vi "spectrometer-control.vi"(0 "Value Indicators Input":T3, 5 "Values changed":bool[](array[boolean]), 7 "Spectrograph Reset Input":T1, 8 "Reset Indicators after Init/Loop":T2, 9 "Spectrograph Value Input":T4={"Slit Width (µm)"=50.0, "Diffraction Grating"=3, "Central Wavelength (nm)"=1000.0, "Filter"=4, "Shutter"=0} {"Shutter" items=["Close", "Open"]; "Slit Width (µm)" min=10.0 max=2500.0 step=0.1 format="%.1f"; "Diffraction Grating" items=["150 lines/mm, 500 nm blaze"=1, "150 lines/mm, 800 nm blaze"=2, "150 lines/mm, 1250 nm blaze"=3]; "Filter" items=["Empty"=5, "Longpass 900 nm"=4, "Longpass 715 nm"=3, "Longpass 475 nm"=2, "Longpass 320 nm"=1]; "Central Wavelength (nm)" min=200.0 max=2000.0 step=0.1 format="%.1f"}) -> (1 "Reset Indicators":T2, 2 "Value Indicators Output":T3, 3 "Spectrograph Value Output":T4={"Slit Width (µm)"=50.0, "Diffraction Grating"=3, "Central Wavelength (nm)"=1000.0, "Filter"=4, "Shutter"=0} {"Shutter" items=["Close", "Open"]; "Slit Width (µm)" min=10.0 max=2500.0 step=0.1 format="%.1f"; "Diffraction Grating" items=["150 lines/mm, 500 nm blaze"=1, "150 lines/mm, 800 nm blaze"=2, "150 lines/mm, 1250 nm blaze"=3]; "Filter" items=["Empty"=5, "Longpass 900 nm"=4, "Longpass 715 nm"=3, "Longpass 475 nm"=2, "Longpass 320 nm"=1]; "Central Wavelength (nm)" min=200.0 max=2000.0 step=0.1 format="%.1f"}, 4 "Spectrograph Reset Output":T1)   [LabVIEW 2015]
uses:
  <userlib>/Shamrock.llb/shamrock_autoSlit_typedef.ctl
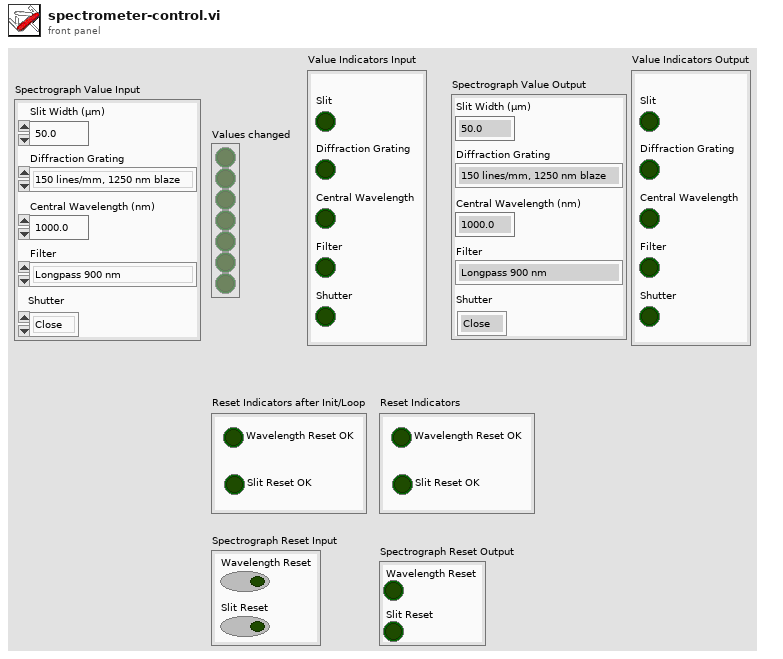
[diagram p1: front panel]
types:
  T1 = cluster{"Wavelength Reset":bool, "Slit Reset":bool}
  T2 = cluster{"Wavelength Reset OK":bool, "Slit Reset OK":bool}
  T3 = cluster{"Slit":bool, "Diffraction Grating":bool, "Central Wavelength":bool, "Filter":bool, "Shutter":bool}
  T4 = cluster{"Slit Width (µm)":dbl, "Diffraction Grating":u16, "Central Wavelength (nm)":dbl, "Filter":u16, "Shutter":u16}
  T5 = typedef "shamrock_autoSlit_typedef.ctl" = enum32{"Reserved (0)", "INPUT SIDE", "INPUT DIRECT", "OUTPUT SIDE", "OUTPUT DIRECT"}
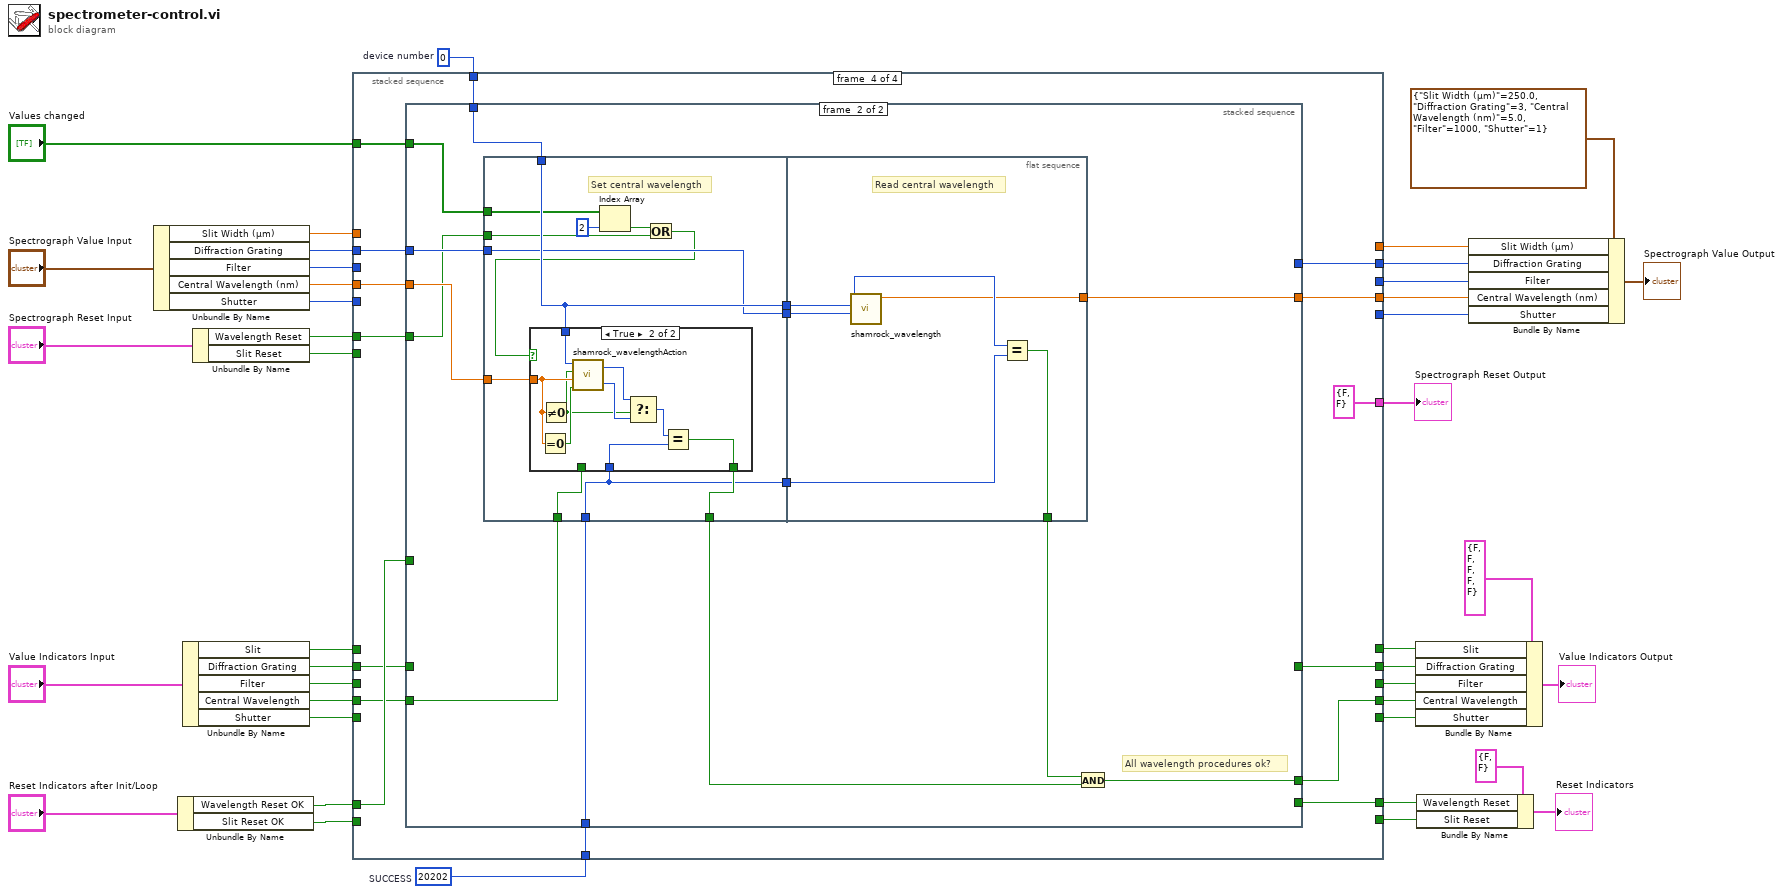
[diagram p0: block diagram]
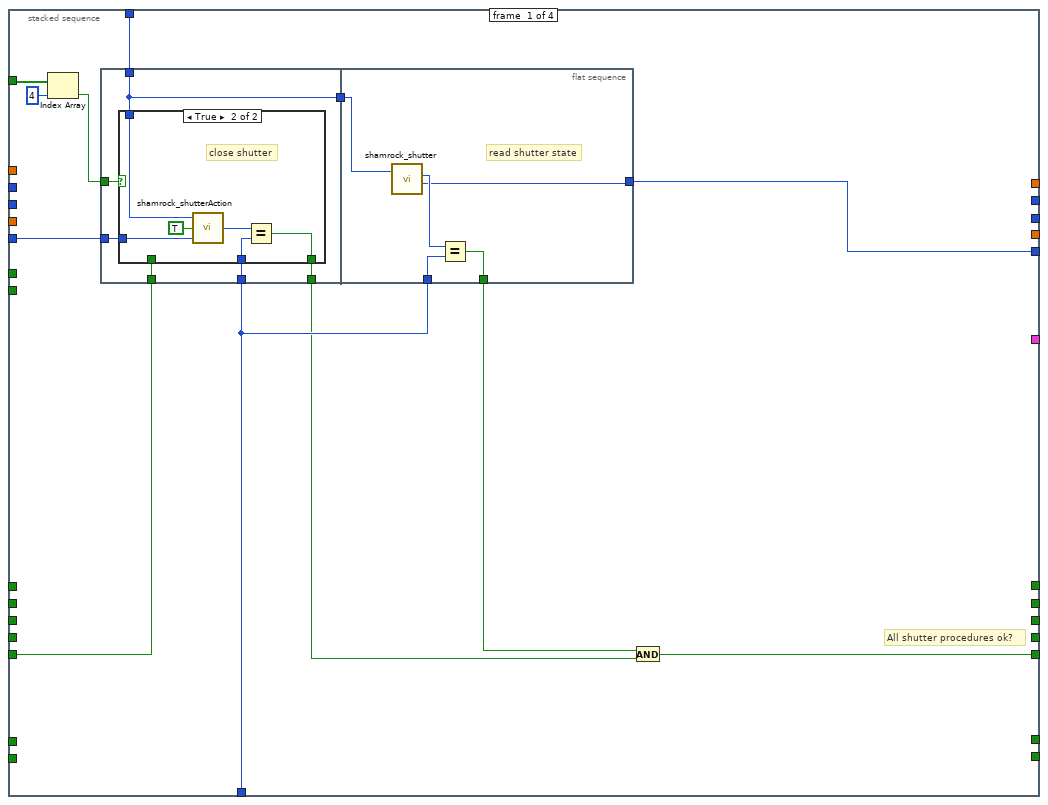
[diagram p2: hidden frame]
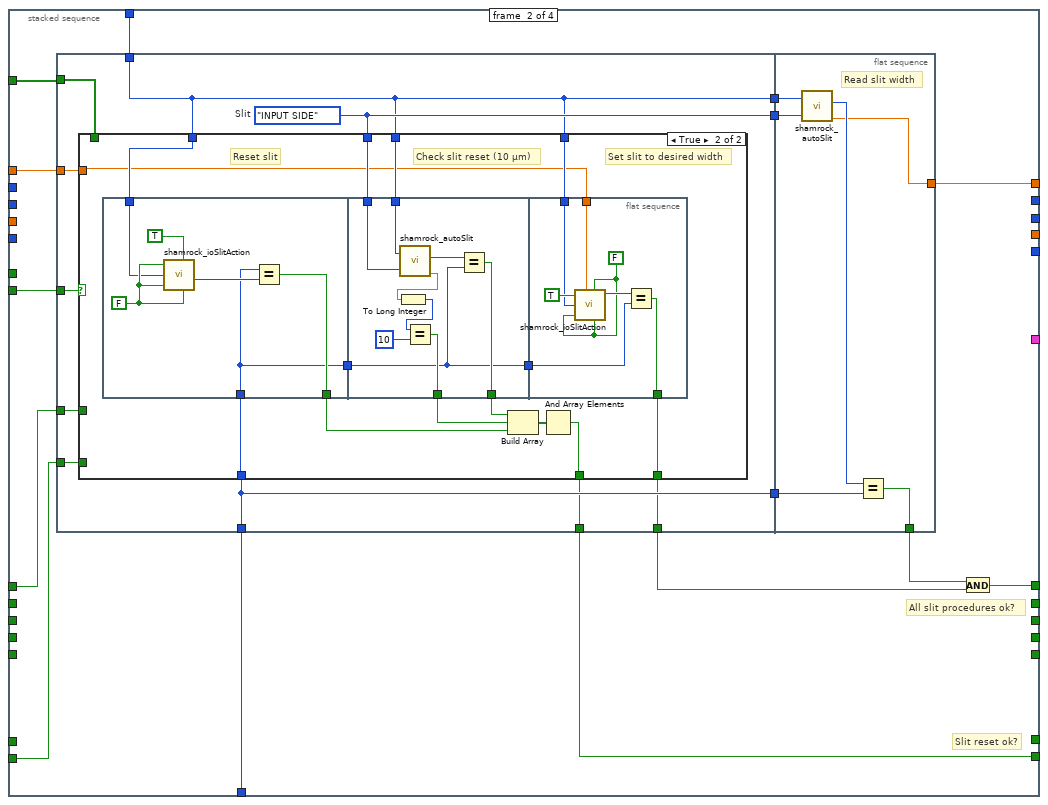
[diagram p4: hidden frame]
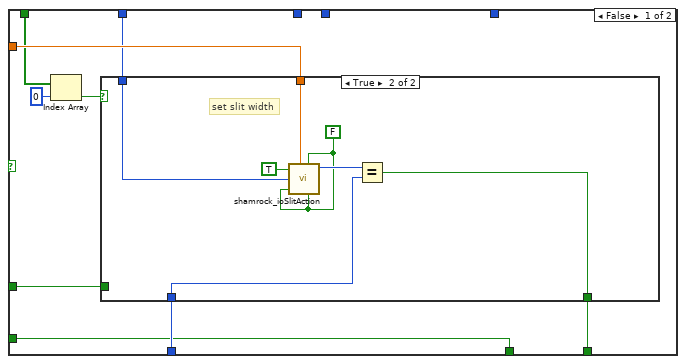
[diagram p5: hidden frame]
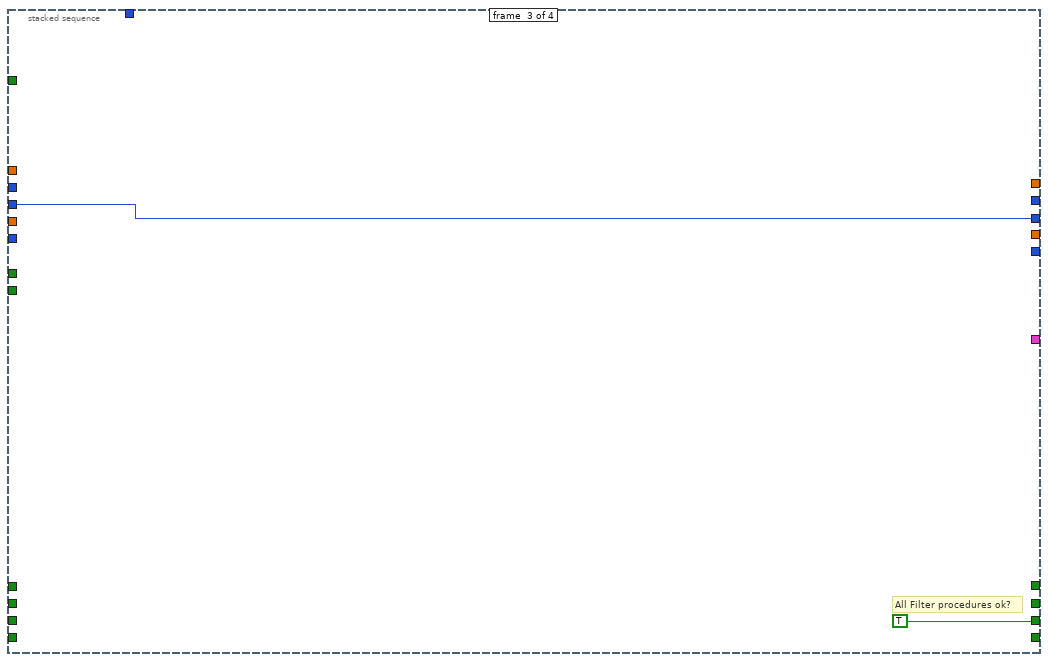
[diagram p7: hidden frame]
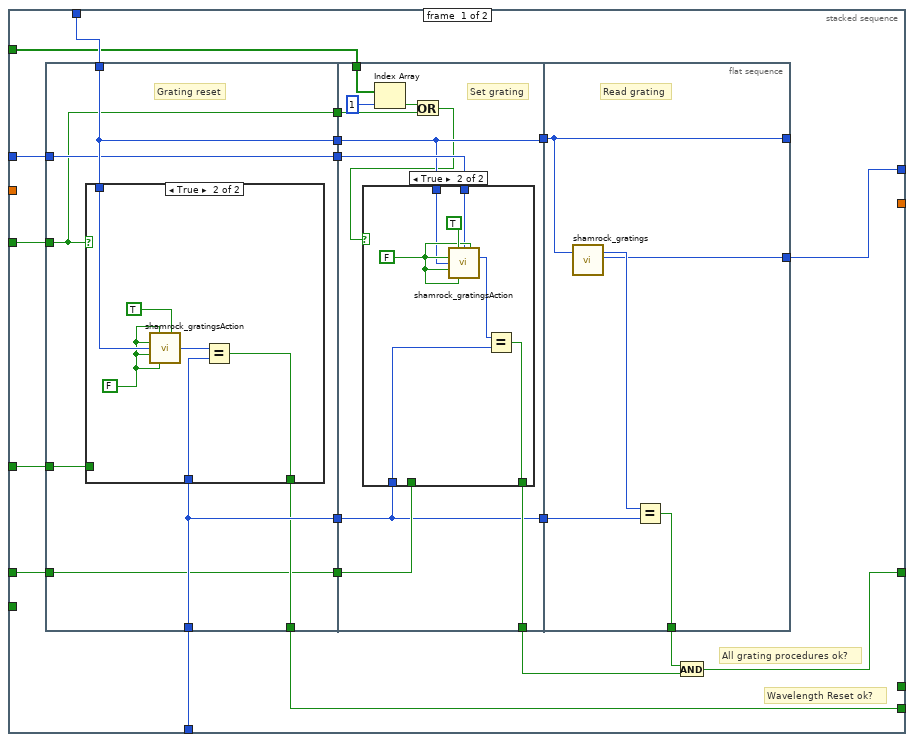
[diagram p8: hidden frame]
diagram:
  w4 = 20202  # SUCCESS
  w5 = 0  # device number
  n1 = Unbundle By Name("Spectrograph Value Input") -> ("Slit Width (µm)"=w40:dbl, "Diffraction Grating"=w39:u16, "Filter"=w36:u16, "Central Wavelength (nm)"=w32:dbl, "Shutter"=w31:u16)
  n2 = Unbundle By Name("Reset Indicators after Init/Loop") -> ("Wavelength Reset OK"=w15:bool, "Slit Reset OK"=w13:bool)
  n3 = Unbundle By Name("Value Indicators Input") -> ("Slit"=w12:bool, "Diffraction Grating"=w8:bool, "Filter"=w11:bool, "Central Wavelength"=w10:bool, "Shutter"=w9:bool)
  n4 = Unbundle By Name("Spectrograph Reset Input") -> ("Wavelength Reset"=w38:bool, "Slit Reset"=w37:bool)
  n5 = stacked-sequence {
    tunnel: w40 -> [_ w84 _ _]
    tunnel: w39 -> [_ _ _ w166]
    tunnel: w38 -> [_ _ _ w169]
    tunnel: w36 -> [_ _ w156 _]
    tunnel: w37 -> [_ w83 _ _]
    tunnel: w31 -> [w50 _ _ _]
    tunnel: w32 -> [_ _ _ w167]
    tunnel: w5 -> [w52 w82 _ w170]
    tunnel: w4 -> [w49 w85 _ w171]
    tunnel: [_ w79 _ _] -> w35
    tunnel: [w46 _ _ _] -> w23
    tunnel: [_ w73 _ _] -> w25
    tunnel: [_ _ TRUE _] -> w24
    tunnel: [_ _ _ w168] -> w27
    tunnel: [_ _ _ w165] -> w34
    tunnel: [_ _ _ w164] -> w26
    tunnel: [w45 _ _ _] -> w33
    tunnel: [_ _ w156 _] -> w20
    tunnel: "Values changed" -> [w44 w75 _ w163]
    tunnel: [_ _ _ w162] -> w28
    tunnel: [_ w77 _ _] -> w29
    tunnel: w15 -> [_ _ _ w161]
    tunnel: w12 -> [_ w76 _ _]
    tunnel: w9 -> [w42 _ _ _]
    tunnel: w11 -> [_ _ _ _]
    tunnel: w8 -> [_ _ _ w160]
    tunnel: w10 -> [_ _ _ w159]
    tunnel: [_ _ _ w158] -> w19
    tunnel: [_ _ _ T1 {"Wavelength Reset"=FALSE, "Slit Reset"=FALSE} ("Spectrograph Reset Output")] -> w7
    tunnel: w13 -> [_ w74 _ _]
    frame #0 {
      # "All shutter procedures ok?"
      n6 = Index Array(array=w44, index=4) -> (element=w41:bool)
      n7 = flat-sequence {
        tunnel: [w58] -> w47
        tunnel: w52 -> [w57]
        tunnel: [w57] -> w51
        tunnel: w50 -> [w55]
        tunnel: w49 -> [w56]
        tunnel: w41 -> [w54]
        tunnel: w42 -> [w53]
        tunnel: w51 -> [w66]
        tunnel: w49 -> [w70]
        tunnel: [w69] -> w48
        tunnel: [w67] -> w45
        frame #0 {
          n8 = case shown="True" w54 {
            tunnel: [w59 w64] -> w58
            tunnel: w57 -> [_ w63]
            tunnel: w56 -> [_ w61]
            tunnel: w55 -> [_ w60]
            tunnel: w53 -> [w59 _]
            frame False {
            }
            frame True {
              # "close shutter"
              n9 = call <userlib>:"shamrock_shutterAction.vi"("Mode"=w60, "SetShutter"=TRUE, "Device No"=w63) -> ("SetShutter"=w62:u32)
              n10 = Equal?(x=w62, y=w61) -> (x = y?=w64:bool)
            }
          }
        }
        frame #1 {
          # "read shutter state"
          n11 = call <userlib>:"shamrock_shutter.vi"("Device No"=w66) -> ("GetShutter"=w68:u32, "Shutter"=w67:i32)  [unwired: 1 in, 4 out]
          n12 = Equal?(x=w68, y=w70) -> (x = y?=w69:bool)
        }
      }
      n13 = And(x=w48, y=w47) -> (x .and. y?=w46:bool)
    }
    frame #1 {
      # "Slit reset ok?"
      # "All slit procedures ok?"
      n14 = flat-sequence {
        tunnel: w85 -> [w92]
        tunnel: w84 -> [w94]
        tunnel: w83 -> [w93]
        tunnel: w82 -> [w88]
        tunnel: [w95] -> w81
        tunnel: [w92] -> w80
        tunnel: [w88] -> w78
        tunnel: [w91] -> w77
        tunnel: [w90] -> w71
        tunnel: w76 -> [w87]
        tunnel: w75 -> [w89]
        tunnel: w74 -> [w86]
        tunnel: w81 -> [w151]
        tunnel: [w153] -> w72
        tunnel: w80 -> [w149]
        tunnel: [w152] -> w79
        tunnel: w78 -> [w150]
        frame #0 {
          w95 = shamrock_autoSlit_typedef."INPUT SIDE"  # Slit
          n15 = case shown="True" w93 {
            tunnel: w88 -> [w103 w124]
            tunnel: w95 -> [_ w122]
            tunnel: w92 -> [w102 w123]
            tunnel: w94 -> [w104 w114]
            tunnel: w88 -> [_ w121]
            tunnel: w88 -> [_ w120]
            tunnel: w89 -> [w100 _]
            tunnel: [w96 w116] -> w91
            tunnel: [w98 w115] -> w90
            tunnel: w87 -> [w97 _]
            tunnel: w86 -> [w96 _]
            frame False {
              n16 = Index Array(array=w100, index=0) -> (element=w99:bool)
              n17 = case shown="True" w99 {
                tunnel: [w105 w106] -> w98
                tunnel: w104 -> [_ w109]
                tunnel: w103 -> [_ w108]
                tunnel: w102 -> [_ w107]
                tunnel: w97 -> [w105 _]
                frame False {
                }
                frame True {
                  w111 = FALSE ("Reset Slit")
                  # "set slit width"
                  n18 = call <userlib>:"shamrock_ioSlitAction.vi"("SetSlit"=TRUE, "Slit Width"=w109, "Device No"=w108, "SetOuputSlit"=w111, "Reset Slit"=w111, "Reset Output Slit"=w111) -> ("SetSlit"=w112:u32)  [unwired: 1 in, 3 out]
                  n19 = Equal?(x=w112, y=w107) -> (x = y?=w106:bool)
                }
              }
            }
            frame True {
              # "Set slit to desired width"
              # "Check slit reset (10 µm)"
              # "Reset slit"
              n20 = flat-sequence {
                tunnel: [w129] -> w119
                tunnel: [w127] -> w126
                tunnel: w124 -> [w128]
                tunnel: w123 -> [w127]
                tunnel: [w137] -> w118
                tunnel: [w136] -> w113
                tunnel: [w135] -> w125
                tunnel: w126 -> [w135]
                tunnel: w122 -> [w134]
                tunnel: w120 -> [w133]
                tunnel: w125 -> [w145]
                tunnel: [w142] -> w115
                tunnel: w121 -> [w144]
                tunnel: w114 -> [w143]
                frame #0 {
                  w131 = FALSE ("SetSlit")
                  n21 = call <userlib>:"shamrock_ioSlitAction.vi"("SetSlit"=w131, "Device No"=w128, "SetOuputSlit"=w131, "Reset Slit"=TRUE, "Reset Output Slit"=w131) -> ("ResetSlit"=w130:u32)  [unwired: 2 in, 3 out]
                  n22 = Equal?(x=w127, y=w130) -> (x = y?=w129:bool)
                }
                frame #1 {
                  n23 = call <userlib>:"shamrock_autoSlit.vi"("Device No"=w133, "Slit"=w134) -> ("RC_GetSlit"=w138:u32, "Slit width (mm)"=w140:dbl)  [unwired: 2 out]
                  n24 = To Long Integer(number=w140) -> (32bit integer=w139:i32)
                  n25 = Equal?(x=w139, y=10) -> (x = y?=w137:bool)
                  n26 = Equal?(x=w138, y=w135) -> (x = y?=w136:bool)
                }
                frame #2 {
                  w147 = FALSE ("Reset Slit")
                  n27 = call <userlib>:"shamrock_ioSlitAction.vi"("SetSlit"=TRUE, "Slit Width"=w143, "Device No"=w144, "SetOuputSlit"=w147, "Reset Slit"=w147, "Reset Output Slit"=w147) -> ("SetSlit"=w148:u32)  [unwired: 1 in, 3 out]
                  n28 = Equal?(x=w148, y=w145) -> (x = y?=w142:bool)
                }
              }
              n29 = Build Array(w113, w118, w119) -> (w117:bool[])
              n30 = And Array Elements(Boolean array=w117) -> (logical AND=w116:bool)
            }
          }
        }
        frame #1 {
          # "Read slit width"
          n31 = call <userlib>:"shamrock_autoSlit.vi"("Device No"=w150, "Slit"=w151) -> ("RC_GetSlit"=w154:u32, "Slit width (mm)"=w152:dbl)  [unwired: 2 out]
          n32 = Equal?(x=w154, y=w149) -> (x = y?=w153:bool)
        }
      }
      n33 = And(x=w72, y=w71) -> (x .and. y?=w73:bool)
    }
    frame #2 {
      # "All Filter procedures ok?"
    }
    frame #3 {
      n34 = stacked-sequence {
        tunnel: w171 -> [w190 w231]
        tunnel: w170 -> [w189 w241]
        tunnel: w169 -> [w186 w229]
        tunnel: [w174 _] -> w168
        tunnel: w167 -> [_ w240]
        tunnel: w166 -> [w184 w237]
        tunnel: [_ w233] -> w165
        tunnel: [_ w232] -> w164
        tunnel: w163 -> [w183 w230]
        tunnel: [w179 _] -> w162
        tunnel: w161 -> [w178 _]
        tunnel: w160 -> [w176 _]
        tunnel: w159 -> [_ w228]
        tunnel: [w175 _] -> w158
        frame #0 {
          # "All grating procedures ok?"
          # "Wavelength Reset ok?"
          n35 = flat-sequence {
            tunnel: w190 -> [w196]
            tunnel: w189 -> [w197]
            tunnel: [w197] -> w188
            tunnel: [w196] -> w187
            tunnel: w186 -> [w193]
            tunnel: [w195] -> w179
            tunnel: [w194] -> w185
            tunnel: w184 -> [w194]
            tunnel: [w193] -> w182
            tunnel: w178 -> [w192]
            tunnel: [w191] -> w177
            tunnel: w176 -> [w191]
            tunnel: w188 -> [w212]
            tunnel: w187 -> [w205]
            tunnel: [w214] -> w173
            tunnel: w185 -> [w213]
            tunnel: w183 -> [w211]
            tunnel: w182 -> [w209]
            tunnel: [w212] -> w181
            tunnel: [w205] -> w180
            tunnel: w177 -> [w206]
            tunnel: [w226] -> _
            tunnel: w181 -> [w226]
            tunnel: w180 -> [w225]
            tunnel: [w224] -> w172
            tunnel: [w223] -> w175
            frame #0 {
              # "Grating reset"
              n36 = case shown="True" w193 {
                tunnel: w197 -> [_ w203]
                tunnel: w196 -> [_ w202]
                tunnel: [w198 w199] -> w195
                tunnel: w192 -> [w198 _]
                frame False {
                }
                frame True {
                  w201 = FALSE ("SetTurret")
                  n37 = call <userlib>:"shamrock_gratingsAction.vi"("WavelengthReset"=TRUE, "SetGrating"=w201, "SetGratingOffset"=w201, "SetTurret"=w201, "Device No"=w203, "SetDetectorOffset"=w201) -> ("WavelengthReset"=w204:u32)  [unwired: 5 in, 4 out]
                  n38 = Equal?(x=w204, y=w202) -> (x = y?=w199:bool)
                }
              }
            }
            frame #1 {
              # "Set grating"
              n39 = Index Array(array=w211, index=1) -> (element=w210:bool)
              n40 = Or(x=w210, y=w209) -> (x .or. y?=w208:bool)
              n41 = case shown="True" w208 {
                tunnel: [w215 w219] -> w214
                tunnel: w213 -> [_ w218]
                tunnel: w212 -> [_ w217]
                tunnel: w206 -> [w215 _]
                tunnel: w205 -> [_ w216]
                frame False {
                }
                frame True {
                  w220 = FALSE ("SetTurret")
                  n42 = call <userlib>:"shamrock_gratingsAction.vi"("WavelengthReset"=w220, "Grating"=w218, "SetGrating"=TRUE, "SetGratingOffset"=w220, "SetTurret"=w220, "Device No"=w217, "SetDetectorOffset"=w220) -> ("SetGrating"=w221:u32)  [unwired: 4 in, 4 out]
                  n43 = Equal?(x=w221, y=w216) -> (x = y?=w219:bool)
                }
              }
            }
            frame #2 {
              # "Read grating"
              n44 = call <userlib>:"shamrock_gratings.vi"("Device No"=w226) -> ("GetGrating"=w227:u32, "Grating"=w223:i32)  [unwired: 2 in, 15 out]
              n45 = Equal?(x=w227, y=w225) -> (x = y?=w224:bool)
            }
          }
          n46 = And(x=w172, y=w173) -> (x .and. y?=w174:bool)
        }
        frame #1 {
          # "All wavelength procedures ok?"
          n47 = flat-sequence {
            tunnel: w241 -> [w251]
            tunnel: w240 -> [w252]
            tunnel: [w251] -> w239
            tunnel: [w250] -> w238
            tunnel: w237 -> [w250]
            tunnel: [w248] -> w236
            tunnel: [w249] -> w235
            tunnel: w231 -> [w248]
            tunnel: w230 -> [w245]
            tunnel: w229 -> [w244]
            tunnel: w228 -> [w242]
            tunnel: w239 -> [w268]
            tunnel: w238 -> [w267]
            tunnel: w236 -> [w265]
            tunnel: [w264] -> w234
            tunnel: [w263] -> w233
            frame #0 {
              # "Set central wavelength"
              n48 = Index Array(array=w245, index=2) -> (element=w247:bool)
              n49 = Or(x=w247, y=w244) -> (x .or. y?=w243:bool)
              n50 = case shown="True" w243 {
                tunnel: w252 -> [_ w259]
                tunnel: w251 -> [_ w262]
                tunnel: [w253 w261] -> w249
                tunnel: w248 -> [_ w260]
                tunnel: w242 -> [w253 _]
                frame False {
                }
                frame True {
                  n51 = Equal To 0?(x=w259) -> (x = 0?=w258:bool)
                  n52 = Not Equal To 0?(x=w259) -> (x != 0?=w254:bool)
                  n53 = call <userlib>:"shamrock_wavelengthAction.vi"("GoToZeroOrder"=w258, "Wavelength"=w259, "SetWavelength"=w254, "Device No"=w262) -> ("GotoZeroOrder"=w255:u32, "SetWavelength"=w257:u32)
                  n54 = Select(t=w257, s=w254, f=w255) -> (s? t:f=w256:u32)
                  n55 = Equal?(x=w256, y=w260) -> (x = y?=w261:bool)
                }
              }
            }
            frame #1 {
              # "Read central wavelength"
              n56 = call <userlib>:"shamrock_wavelength.vi"("Grating No"=w267, "Device No"=w268) -> ("GetWavelength"=w266:u32, "Wavelength"=w263:dbl)  [unwired: 7 out]
              n57 = Equal?(x=w266, y=w265) -> (x = y?=w264:bool)
            }
          }
          n58 = And(x=w234, y=w235) -> (x .and. y?=w232:bool)
        }
      }
    }
  }
  "Spectrograph Reset Output" <- w7
  n59 = Bundle By Name(cluster=T3 {"Slit"=FALSE, "Diffraction Grating"=FALSE, "Central Wavelength"=FALSE, "Filter"=FALSE, "Shutter"=FALSE} ("Value Indicators Output"), "Slit"=w25, "Diffraction Grating"=w27, "Filter"=w24, "Central Wavelength"=w26, "Shutter"=w23) -> (→"Value Indicators Output":T3)
  n60 = Bundle By Name(cluster=T1 {"Wavelength Reset"=FALSE, "Slit Reset"=FALSE} ("Reset Control Cluster"), "Wavelength Reset"=w28, "Slit Reset"=w29) -> (→"Reset Indicators":T1)
  n61 = Bundle By Name(cluster=T4 {"Slit Width (µm)"=250.0, "Diffraction Grating"=3, "Central Wavelength (nm)"=5.0, "Filter"=1000, "Shutter"=1} ("Spectrograph Value Output"), "Slit Width (µm)"=w35, "Diffraction Grating"=w19, "Filter"=w20, "Central Wavelength (nm)"=w34, "Shutter"=w33) -> (→"Spectrograph Value Output":T4)
